vi "例4.13-7while循环加事件结构 -超时分支（常见问题10）.vi"() -> ()   [LabVIEW 2017]
panel:
  out "和":dbl
  in  "加数2":dbl
  in  "加数1":dbl
  in  "停止":bool
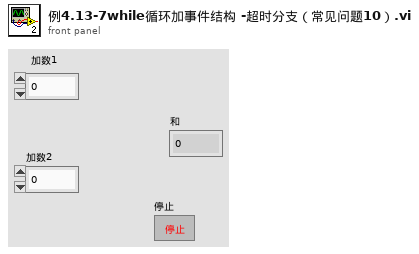
[diagram p1: front panel]
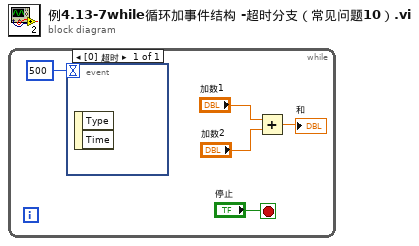
[diagram p0: block diagram]
diagram:
  n1 = while {
    stop <- "停止" stop-if-true
    n2 = event shown="[0] 超时" {
      selector: _ -> [_]
      dyn-events: _ -> [_]
      timeout: 500 -> [_]
      event Timeout {
        n3 = event-data() -> ()  [unwired: 1 in, 2 out]
      }
    }
    n4 = Add(x="加数1", y="加数2") -> (x+y=→"和":dbl)
  }
